vi "Close Rendezvous.vi"(8 "error in (no error)":errorcluster, 11 "System Actor in":refnum<class "System Actor.lvclass">) -> (0 "error out":errorcluster, 3 "System Actor out":refnum<class "System Actor.lvclass">)   [LabVIEW 2024, in "System Actor.lvclass"]
uses:
  System Actor.lvclass
  System Actor.lvclass/System Actor.ctl
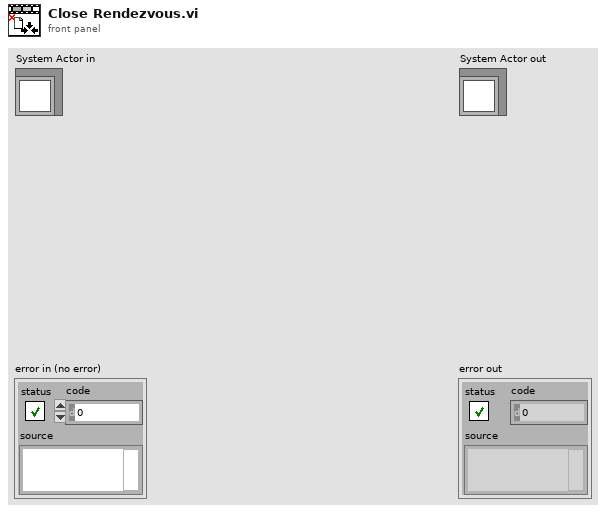
[diagram p1: front panel]
types:
  T1 = typedef "Rendezvous RefNum" = refnum<k1>
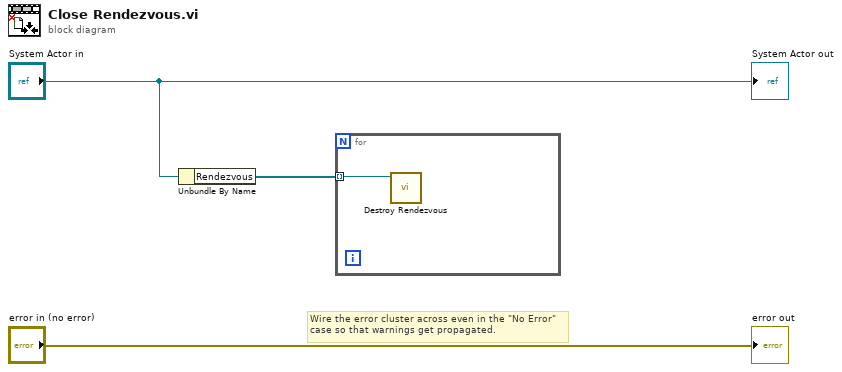
[diagram p0: block diagram]
diagram:
  # "Wire the error cluster across even in the \"No Error\"\ncase so that warnings get propagated."
  n1 = Unbundle By Name("System Actor in") -> ("Rendezvous"=w1:T1[])
  n2 = for {
    tunnel: w1 -> [w4] mode=indexing
    n3 = call <vilib>:"Destroy Rendezvous.vi"("rendezvous"=w4) -> ()  [unwired: 5 in, 2 out]
  }
  "error out" <- "error in (no error)"
  "System Actor out" <- "System Actor in"
